vi "VI task manager.vi"() -> ()   [LabVIEW 2014]
uses:
  <vilib>/Utility/cursorutil.llb/Set Cursor (Icon Pict).vi
panel:
  in  "Show:":T1(ring)
  in  "ShowFP":bool
  in  "AbortEx":bool
  in  "stop":bool
  out "VIs":string[][](table)
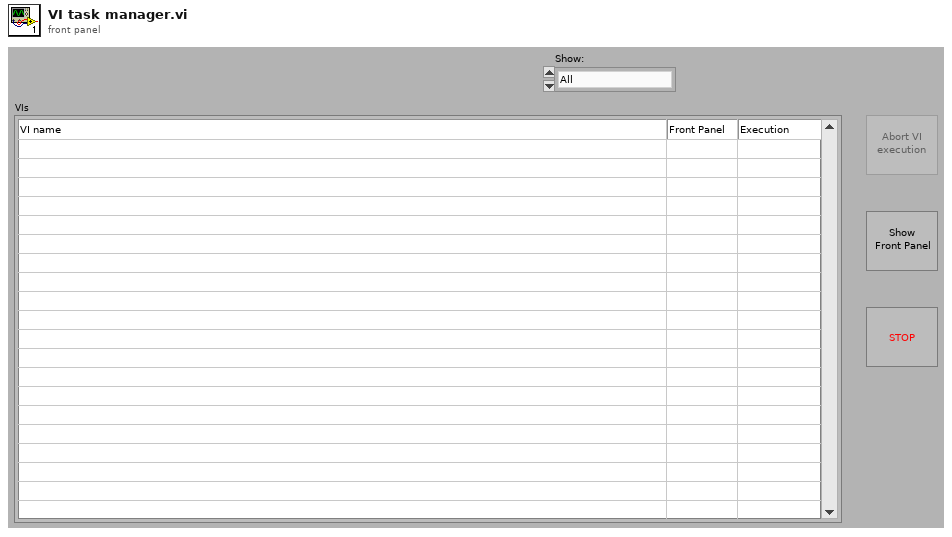
[diagram p1: front panel]
types:
  T1 = enum32{"All", "Bad", "Idle", "Run top level", "Running"}
  T2 = enum32{"Invalid", "Standard", "Closed", "Hidden", "Minimized", "Maximized"}
  T3 = enum32{"Bad", "Idle", "Run top level", "Running"}
  T4 = typedef "LVRowAndColumnTypeDef.ctl" = cluster{"Row":i32, "Column":i32}
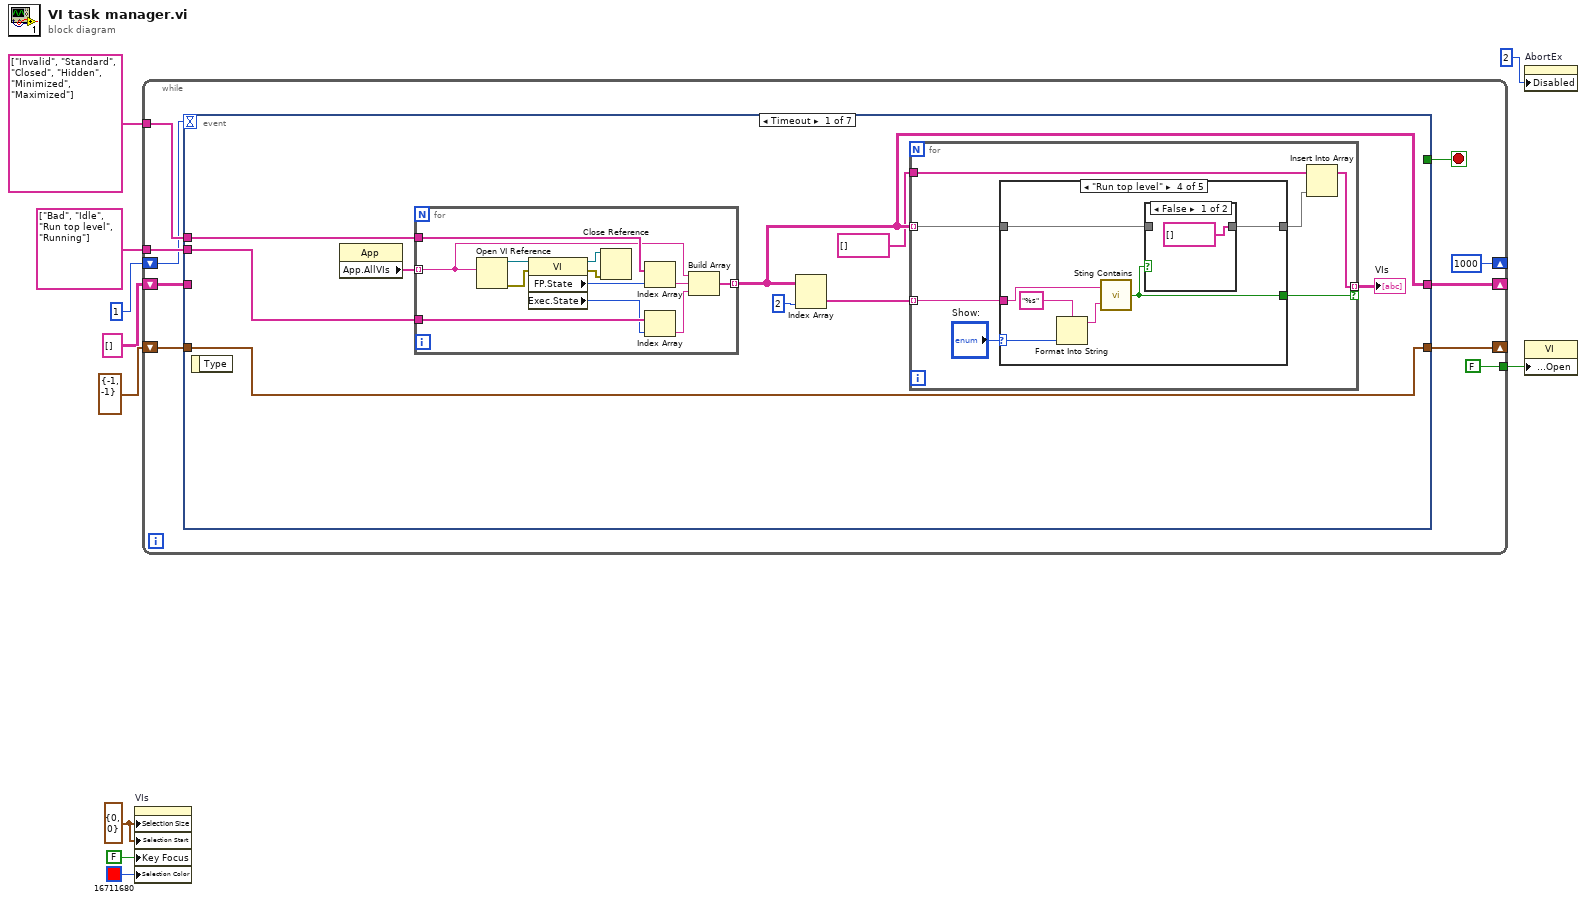
[diagram p0: block diagram]
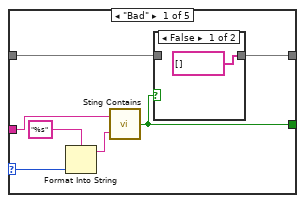
[diagram p2: hidden frame]
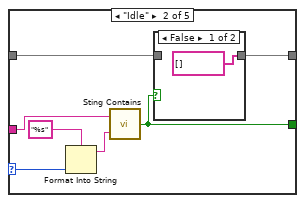
[diagram p4: hidden frame]
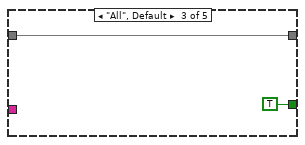
[diagram p6: hidden frame]
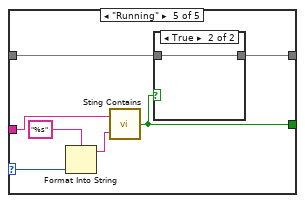
[diagram p8: hidden frame]
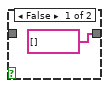
[diagram p9: hidden frame]
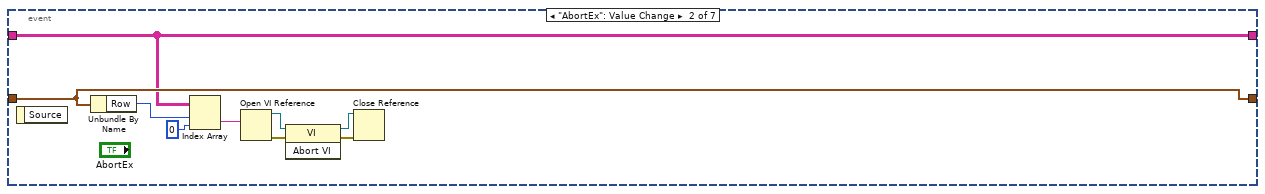
[diagram p10: hidden frame]
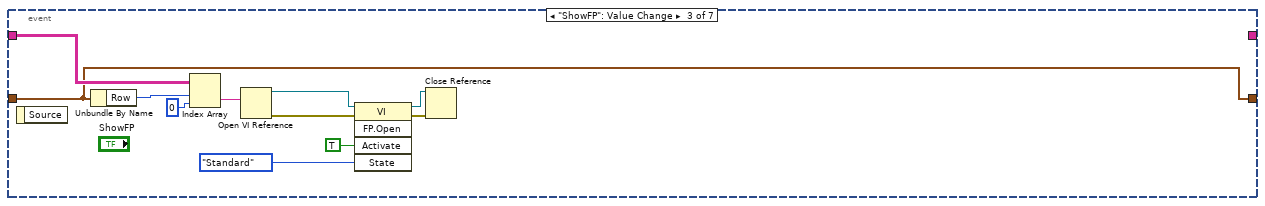
[diagram p11: hidden frame]
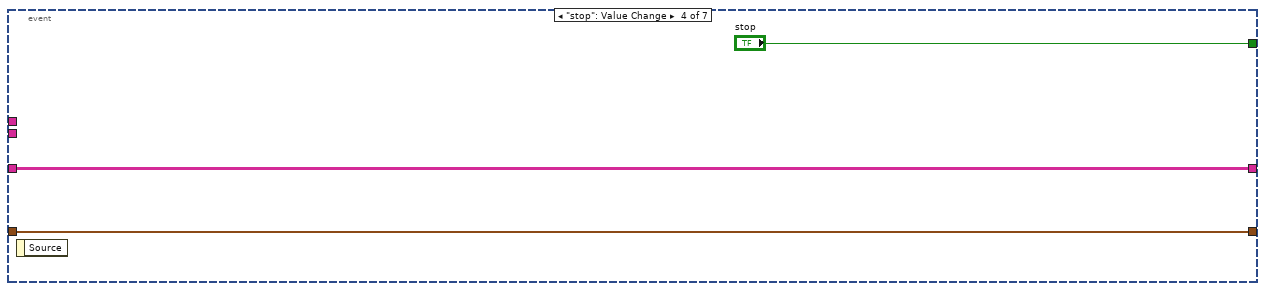
[diagram p12: hidden frame]
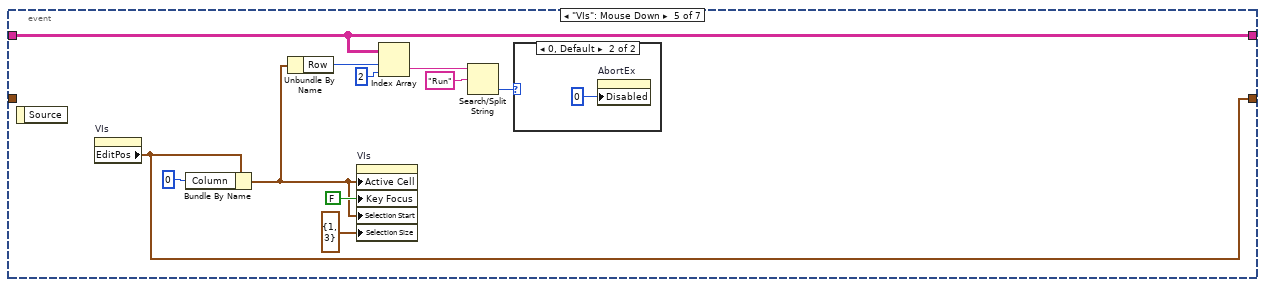
[diagram p13: hidden frame]
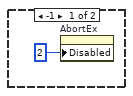
[diagram p14: hidden frame]
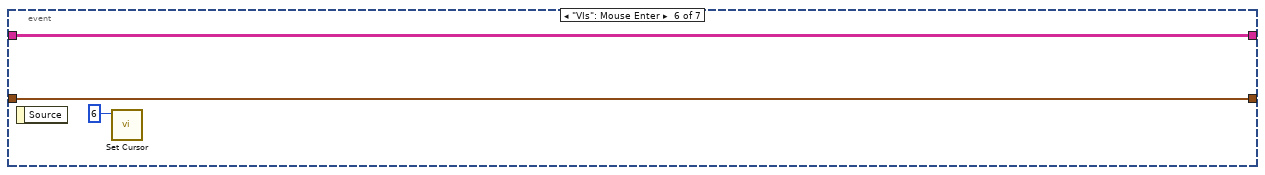
[diagram p15: hidden frame]
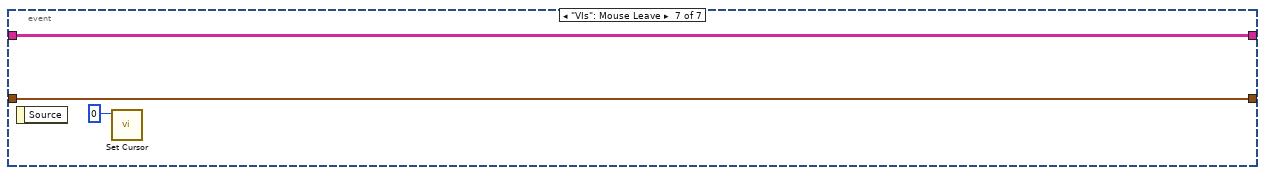
[diagram p16: hidden frame]
diagram:
  w2 = cluster{"Row":i32, "Column":i32} {"Row"=0, "Column"=0} ("Active Cell:Active Cell")
  n1 = property on="VIs" class="Tbl (strict)"("Selection Size"=w2, "Selection Start"=w2, "Key Focus"=FALSE, "Selection Color"=u32 16711680) -> ()  [unwired: 2 in, 2 out]
  n2 = while {
    tunnel: string[] ["Bad", "Idle", "Run top level", "Running"] ("Application:All VIs In Memory") -> [w20]
    tunnel: string[] ["Invalid", "Standard", "Closed", "Hidden", "Minimized", "Maximized"] ("Strings []") -> [w19]
    shift-right: [1000] -> _
    shift-left: 1 -> [w17]
    shift-right: [w16] -> _
    shift-left: cluster{"Row":i32, "Column":i32} {"Row"=-1, "Column"=-1} ("EditPos") -> [w15]
    shift-right: [w14] -> _
    shift-left: string[][] [] -> [w13]
    tunnel: [FALSE ("stop")] -> w1
    stop <- w12 stop-if-true
    n3 = event shown="[0] Timeout" {
      selector: _ -> [_ _ _ _ _ _ _]
      dyn-events: _ -> [_ _ _ _ _ _ _]
      timeout: w17 -> [_ _ _ _ _ _ _]
      tunnel: w20 -> [w28 _ _ _ _ _ _]
      tunnel: w19 -> [w27 _ _ _ _ _ _]
      tunnel: [_ _ _ "stop" _ _ _] -> w12
      tunnel: [w26 w93 w98 w108 w119 w124 w127] -> w16
      tunnel: w15 -> [w26 w93 w98 w108 _ w124 w127]
      tunnel: [w23 w92 _ w107 w110 w123 w126] -> w14
      tunnel: w13 -> [_ w92 w99 w107 w110 w123 w126]
      event Timeout {
        n4 = event-data() -> ()  [unwired: 1 in, 1 out]
        n5 = property class="App"() -> ("App.AllVIs"=w29:string[])  [unwired: 2 in, 2 out]
        n6 = for {
          tunnel: w29 -> [w81] mode=indexing
          tunnel: w28 -> [w86]
          tunnel: w27 -> [w82]
          tunnel: [w78] -> w23 mode=indexing
          n7 = Open VI Reference(vi path=w81) -> (vi reference=w75:refnum<vi>, error out=w84:errorcluster)  [unwired: 5 in]
          n8 = property class="VI"(reference=w75, error in=w84) -> (reference out=w85:refnum<vi>, error out=w83:errorcluster, "FP.State"=w77:T2, "Exec.State"=w76:T3)
          n9 = Close Reference(reference=w85, error in (no error)=w83) -> ()  [unwired: 1 out]
          n10 = Index Array(array=w82, index=w77) -> (element=w80:string)
          n11 = Index Array(array=w86, index=w76) -> (element=w79:string)
          n12 = Build Array(w81, w80, w79) -> (w78:string[])
        }
        n13 = Index Array(array=w23, index (col)=2 ("disabled index (col)")) -> (element=w24:string[])  [unwired: 1 in]
        n14 = for {
          tunnel: w24 -> [w35] mode=indexing
          tunnel: w23 -> [w34] mode=indexing
          tunnel: string[] [] -> [w33]
          tunnel: [w31] -> w22 mode=indexing if=w30
          n15 = case shown="\"Run top level\"" "Show:" {
            selector: "Show:" -> [w43 w49 _ w60 w69]
            tunnel: w35 -> [w41 w50 _ w61 w70]
            tunnel: w34 -> [w39 w48 w56 w59 w68]
            tunnel: [w38 w47 w56 w58 w67] -> w32
            tunnel: [w37 w46 TRUE ("Boolean") w57 w66] -> w30
            frame "Bad" {
              n16 = Format Into String(format string="%s", w43) -> (resulting string=w40:string)  [unwired: 2 in, 1 out]
              n17 = call "Sting Contains.vi"("Expression to evaluate"=w40, "Input String"=w41) -> ("Boolean"=w37:bool)
              n18 = case shown="False" w37 {
                tunnel: w39 -> [_ w45]
                tunnel: [string[] [] w45] -> w38
                frame False {
                }
                frame True {
                }
              }
            }
            frame "Idle" {
              n19 = Format Into String(format string="%s", w49) -> (resulting string=w51:string)  [unwired: 2 in, 1 out]
              n20 = call "Sting Contains.vi"("Expression to evaluate"=w51, "Input String"=w50) -> ("Boolean"=w46:bool)
              n21 = case shown="False" w46 {
                tunnel: w48 -> [_ w54]
                tunnel: [string[] [] w54] -> w47
                frame False {
                }
                frame True {
                }
              }
            }
            frame "All", Default {
            }
            frame "Run top level" {
              n22 = Format Into String(format string="%s", w60) -> (resulting string=w62:string)  [unwired: 2 in, 1 out]
              n23 = call "Sting Contains.vi"("Expression to evaluate"=w62, "Input String"=w61) -> ("Boolean"=w57:bool)
              n24 = case shown="False" w57 {
                tunnel: w59 -> [_ w65]
                tunnel: [string[] [] w65] -> w58
                frame False {
                }
                frame True {
                }
              }
            }
            frame "Running" {
              n25 = Format Into String(format string="%s", w69) -> (resulting string=w71:string)  [unwired: 2 in, 1 out]
              n26 = call "Sting Contains.vi"("Expression to evaluate"=w71, "Input String"=w70) -> ("Boolean"=w66:bool)
              n27 = case shown="True" w66 {
                tunnel: w68 -> [_ w74]
                tunnel: [string[] [] w74] -> w67
                frame False {
                }
                frame True {
                }
              }
            }
          }
          n28 = Insert Into Array(array=w33, new element=w32) -> (w31:string[])  [unwired: 1 in]
        }
        "VIs" <- w22
      }
      event "AbortEx": Value Change {
        n29 = event-data() -> ()  [unwired: 1 in, 1 out]
        n30 = Unbundle By Name(w93) -> ("Row"=w95:i32)
        n31 = Index Array(array=w92, index (row)=w95, index (col)=0 ("disabled index (col)")) -> (element=w87:string)
        n32 = Open VI Reference(vi path=w87) -> (vi reference=w91:refnum<vi>, error out=w89:errorcluster)  [unwired: 5 in]
        n33 = invoke class="VI" method="Abort VI"(reference=w91, error in=w89) -> (reference out=w90:refnum<vi>, error out=w88:errorcluster)  [unwired: 1 in, 1 out]
        n34 = Close Reference(reference=w90, error in (no error)=w88) -> ()  [unwired: 1 out]
      }
      event "ShowFP": Value Change {
        n35 = event-data() -> ()  [unwired: 1 in, 1 out]
        n36 = Unbundle By Name(w98) -> ("Row"=w106:i32)
        n37 = Index Array(array=w99, index (row)=w106, index (col)=0 ("disabled index (col)")) -> (element=w100:string)
        n38 = Open VI Reference(vi path=w100) -> (vi reference=w104:refnum<vi>, error out=w102:errorcluster)  [unwired: 5 in]
        n39 = invoke class="VI" method="FP.Open"(reference=w104, error in=w102, "Activate"=TRUE ("Activate?"), "State"=T2."Standard") -> (reference out=w103:refnum<vi>, error out=w101:errorcluster)  [unwired: 1 in, 3 out]
        n40 = Close Reference(reference=w103, error in (no error)=w101) -> ()  [unwired: 1 out]
      }
      event "stop": Value Change {
        n41 = event-data() -> ()  [unwired: 1 in, 1 out]
      }
      event "VIs": Mouse Down {
        n42 = event-data() -> ()  [unwired: 1 in, 1 out]
        n43 = property on="VIs" class="Tbl (strict)"() -> ("EditPos"=w119:T4)  [unwired: 2 in, 2 out]
        n44 = Bundle By Name(cluster=w119, "Column"=0) -> (w116:T4)
        n45 = Unbundle By Name(w116) -> ("Row"=w115:i32)
        n46 = property on="VIs" class="Tbl (strict)"("Active Cell"=w116, "Key Focus"=FALSE, "Selection Start"=w116, "Selection Size"=cluster{"Row":i32, "Column":i32} {"Row"=1, "Column"=3}) -> ()  [unwired: 2 in, 2 out]
        n47 = Index Array(array=w110, index (row)=w115, index (col)=2 ("disabled index (col)")) -> (element=w113:string)
        n48 = Search/Split String(string=w113, search string/char (-)="Run") -> (offset of match=w111:i32)  [unwired: 1 in, 2 out]
        n49 = case shown="0, Default" w111 {
          frame -1 {
            n50 = property on="AbortEx" class="Bool"("Disabled"=u8 2) -> ()  [unwired: 2 in, 2 out]
          }
          frame 0, Default {
            n51 = property on="AbortEx" class="Bool"("Disabled"=u8 0) -> ()  [unwired: 2 in, 2 out]
          }
        }
      }
      event "VIs": Mouse Enter {
        n52 = event-data() -> ()  [unwired: 1 in, 1 out]
        n53 = call-poly <vilib>:"Set Cursor.vi"("icon"=u16 6) -> ()  [unwired: 9 in, 2 out]
      }
      event "VIs": Mouse Leave {
        n54 = event-data() -> ()  [unwired: 1 in, 1 out]
        n55 = call-poly <vilib>:"Set Cursor.vi"("icon"=u16 0) -> ()  [unwired: 9 in, 2 out]
      }
    }
  }
  n56 = property on="AbortEx" class="Bool"("Disabled"=u8 2) -> ()  [unwired: 2 in, 2 out]
  n57 = property class="VI"("Front Panel.Open"=w1) -> ()  [unwired: 2 in, 2 out]
